vi "UTILITY Modbus 32bit Number Combine.vi"(10 "Swap Words":bool=TRUE, 11 "Holding Registers":u16[](array[numeric]) format="%.0x") -> (2 "word swapped":u32, 3 "Data":sgl)   [LabVIEW 2020]
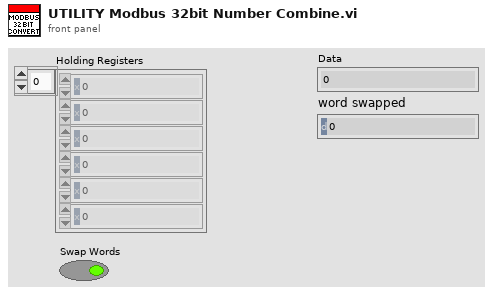
[diagram p1: front panel]
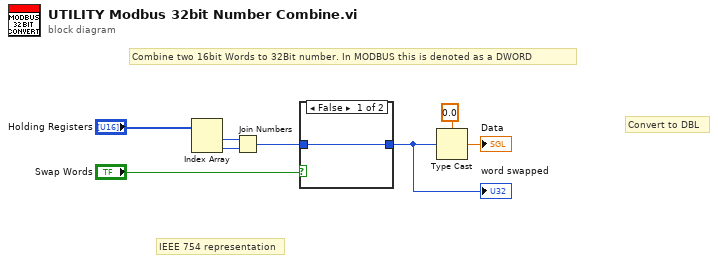
[diagram p0: block diagram]
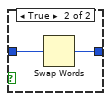
[diagram p2: hidden frame]
diagram:
  # "IEEE 754 representation"
  # "Convert to DBL"
  # "Combine two 16bit Words to 32Bit number. In MODBUS this is denoted as a DWORD"
  n1 = Index Array(array="Holding Registers") -> (element #1=w4:u16, element #2=w5:u16)  [unwired: 2 in]
  n2 = Join Numbers(hi=w4, lo=w5) -> ((hi.lo)=w3:u32)
  n3 = case shown="False" "Swap Words" {
    tunnel: [w9 w11] -> w1
    tunnel: w3 -> [w9 w10]
    frame False {
    }
    frame True {
      n4 = Swap Words(1:w10) -> (0:w11:u32)
    }
  }
  "word swapped" <- w1
  n5 = Type Cast(type=sgl 0.0, x=w1) -> (*(type *) &x=→"Data":sgl)
